vi "display permission to classification.vi"(10 "supported classes":T1[](array[typedef])=[enum."processing parameter", enum."processing result"], 11 "display permissions":T2=enum."Read from Memory") -> (3 "channel classification":T1)   [LabVIEW 2013, in "Shared Memory editor node.lvclass"]
doc: "Converts from the 'display permissions' type-def to the 'channel classification' type-def."
uses:
  Shared Memory editor node.lvclass
  <vilib>/NI/Tag Bus Module Framework/channel/channel classification.ctl
  permissions.ctl
  <vilib>/NI/Tag Bus Module Framework/channel/TBM channel.lvclass
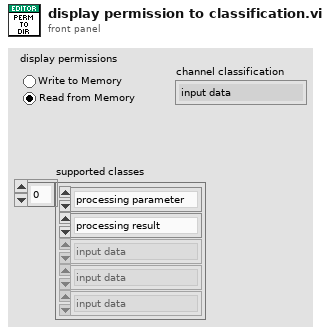
[diagram p1: front panel]
types:
  T1 = typedef "TBM channel.lvclass/channel classification.ctl" = enum16{"input data", "output data", "processing parameter", "processing result"}
  T2 = typedef "Shared Memory editor node.lvclass/permissions.ctl" = enum32{"Write to Memory", "Read from Memory"}
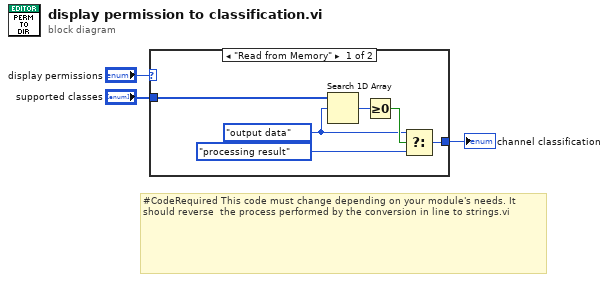
[diagram p0: block diagram]
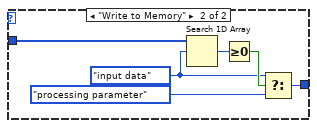
[diagram p2: hidden frame]
diagram:
  # "#CodeRequired This code must change depending on your module's needs. It should reverse  the process performed by the conversion in line to strings.vi"
  n1 = case shown="\"Read from Memory\"" "display permissions" {
    tunnel: [w5 w11] -> w3
    tunnel: "supported classes" -> [w9 w15]
    frame "Read from Memory" {
      w6 = channel_classification."output data" ("channel classification")
      n2 = Search 1D Array(1D array=w9, element=w6) -> (index of element=w8:i32)  [unwired: 1 in]
      n3 = Greater Or Equal To 0?(x=w8) -> (x >= 0?=w7:bool)
      n4 = Select(t=w6, s=w7, f=channel_classification."processing result" ("channel classification")) -> (s? t:f=w5:T1)
    }
    frame "Write to Memory" {
      w12 = channel_classification."input data" ("channel classification")
      n5 = Search 1D Array(1D array=w15, element=w12) -> (index of element=w14:i32)  [unwired: 1 in]
      n6 = Greater Or Equal To 0?(x=w14) -> (x >= 0?=w13:bool)
      n7 = Select(t=w12, s=w13, f=channel_classification."processing parameter" ("channel classification")) -> (s? t:f=w11:T1)
    }
  }
  "channel classification" <- w3
